vi "API - Compile Tx Channel Refs.vi"(6 "Packet Name":string, 7 "Timestamp Present?":bool, 8 "error in (no error)":errorcluster, 11 "Item Ref in":T1 format="%.0x") -> (0 "error out":errorcluster, 2 "Data types":T3[](array[typedef]), 3 "Item Ref out":T1 format="%.0x", 4 "Tx Ref Array":T2 {"VS Refs" format="%.0x"})   [LabVIEW 2016, in "UDP-Custom-Device System Explorer.lvlib"]
uses:
  UDP-Custom-Device System Explorer.lvlib
  Types/Channel Data Type.ctl
  <vilib>/NI Veristand/Custom Device API/Custom Device Item Ref.ctl
  Shared/Constants.vi
  <vilib>/NI VeriStand/Custom Device API/Custom Device API.lvlib
  <vilib>/NI VeriStand/Custom Device Tools/Custom Device Utility Library/Custom Device Utility Library.lvlib
  Shared/UDP-Custom-Device Shared.lvlib
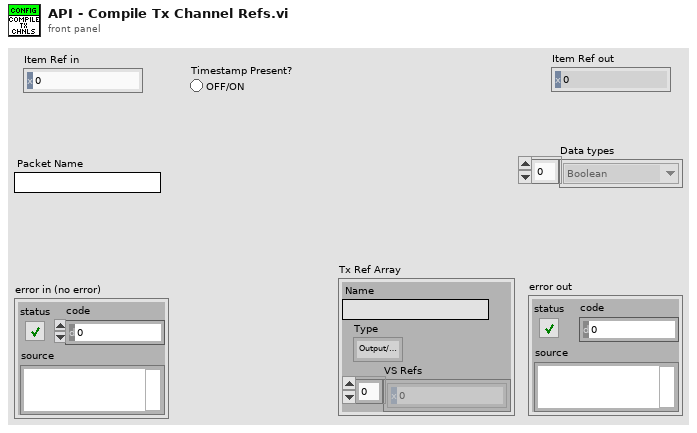
[diagram p1: front panel]
types:
  T1 = typedef "Custom Device API.lvlib/Custom Device Item Ref.ctl" = u64
  T2 = cluster{"Name":string, "Type":enum16{"Output/Write", "Input/Read", "Input/ReadWrite"}, "VS Refs":T1[]}
  T3 = typedef "UDP-Custom-Device Shared.lvlib/Channel Data Type.ctl" = enum16{"Boolean", "Single", "Double", "I8", "I16", "I32", "I64", "U8", "U16", "U32", "U64"}
  T4 = enum16{"Output/Write", "Input/Read", "Input/ReadWrite"}
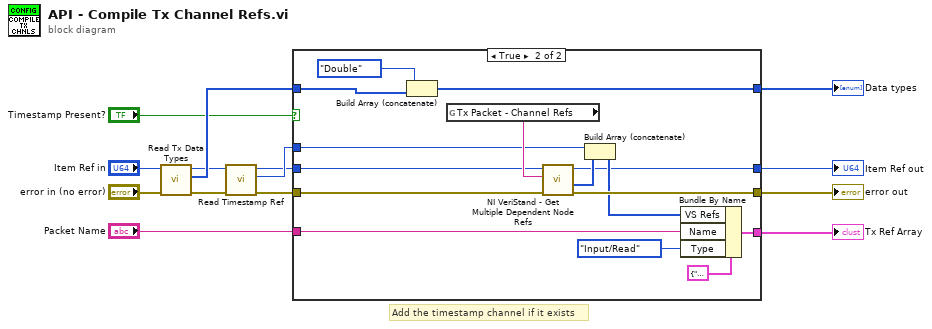
[diagram p0: block diagram]
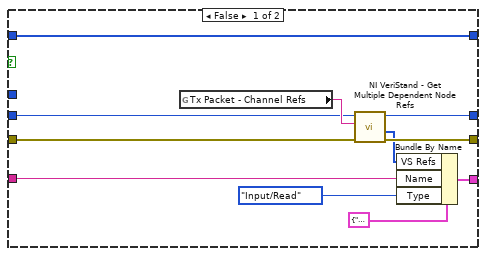
[diagram p2: hidden frame]
diagram:
  # "Add the timestamp channel if it exists"
  n1 = call "Read Tx Data Types.vi"("error in (no error)"="error in (no error)", "Node Ptr"="Item Ref in") -> ("error out"=w9:errorcluster, "Data types"=w13:T3[], "Node Ptr out"=w7:T1)  [unwired: 7 in]
  n2 = call "Read Timestamp Ref.vi"("error in (no error)"=w9, "Node Ptr"=w7) -> ("error out"=w10:errorcluster, "Timestamp Ref"=w12:T1, "Node Ptr out"=w8:T1)  [unwired: 7 in]
  n3 = case shown="True" "Timestamp Present?" {
    tunnel: [w25 w40] -> w2
    tunnel: "Packet Name" -> [w21 w37]
    tunnel: [w19 w35] -> w4
    tunnel: w8 -> [w18 w34]
    tunnel: w10 -> [w17 w33]
    tunnel: w12 -> [_ w32]
    tunnel: w13 -> [w16 w29]
    tunnel: [w16 w28] -> w14
    tunnel: [w15 w26] -> w1
    frame False {
      n4 = global read "Constants.vi" "Tx Packet - Channel Refs"() -> (w24:string)
      n5 = call <vilib>:"NI VeriStand - Get Multiple Dependent Node Refs.vi"("error in (no error)"=w17, "Base Property Name"=w24, "Item Ref in"=w18) -> ("error out"=w25:errorcluster, "Dependent Node Refs"=w22:T1[], "Item Ref out"=w15:T1)  [unwired: 6 in]
      n6 = Bundle By Name(cluster=T2 {"Name"="", "Type"=enum."Output/Write", "VS Refs"=[]} ("Group"), "VS Refs"=w22, "Name"=w21, "Type"=T4."Input/Read") -> (w19:T2)
    }
    frame True {
      n7 = Build Array (concatenate)(Channel_Data_Type."Double" ("element"), w29) -> (w28:T3[])
      n8 = global read "Constants.vi" "Tx Packet - Channel Refs"() -> (w39:string)
      n9 = call <vilib>:"NI VeriStand - Get Multiple Dependent Node Refs.vi"("error in (no error)"=w33, "Base Property Name"=w39, "Item Ref in"=w34) -> ("error out"=w40:errorcluster, "Dependent Node Refs"=w31:T1[], "Item Ref out"=w26:T1)  [unwired: 6 in]
      n10 = Build Array (concatenate)(w32, w31) -> (w30:T1[])
      n11 = Bundle By Name(cluster=T2 {"Name"="", "Type"=enum."Output/Write", "VS Refs"=[]} ("Group"), "VS Refs"=w30, "Name"=w37, "Type"=T4."Input/Read") -> (w35:T2)
    }
  }
  "Data types" <- w14
  "Tx Ref Array" <- w4
  "error out" <- w2
  "Item Ref out" <- w1
